vi "continuous-serial-read.vi"() -> ()   [LabVIEW 2021]
uses:
  <vilib>/regexp/Match Regular Expression.xnode
  <vilib>/Instr/_visa.llb/VISA Configure Serial Port (Instr).vi
  SCD41.ctl
  STC31.ctl
panel:
  in  "state":string
  out "CD5":T1 {"CD3: CO2 (ppm)" format="%.2f"}
  out "CD4":T1 {"CD3: CO2 (ppm)" format="%.2f"}
  out "CD3":T1 {"CD3: CO2 (ppm)" format="%.2f"}
  out "CD2":T2 {"Humidity (%)" format="%.2f"; "Temp (degC)" format="%.2f"; "CO2 (ppm)" format="%.2f"}
  out "CD1":T2 {"Humidity (%)" format="%.2f"; "Temp (degC)" format="%.2f"; "CO2 (ppm)" format="%.2f"}
  out "RHT6: Humidity (%)":dbl format="%.2f"
  out "RHT6: Temp (degC)":dbl format="%.2f"
  out "RHT5: Humidity (%)":dbl format="%.2f"
  out "RHT5: Temp (degC)":dbl format="%.2f"
  out "RHT4: Humidity (%)":dbl format="%.2f"
  out "RHT4: Temp (degC)":dbl format="%.2f"
  out "RHT3: Humidity (%)":dbl format="%.2f"
  out "RHT3: Temp (degC)":dbl format="%.2f"
  out "Num Samples":i32
  out "error out":errorcluster
  out "data string array":string[](array[string])
  out "read buffer":string
  out "Bytes Returned":u32
  in  "VISA resource name":refnum<visa-resource-name>="COM22"
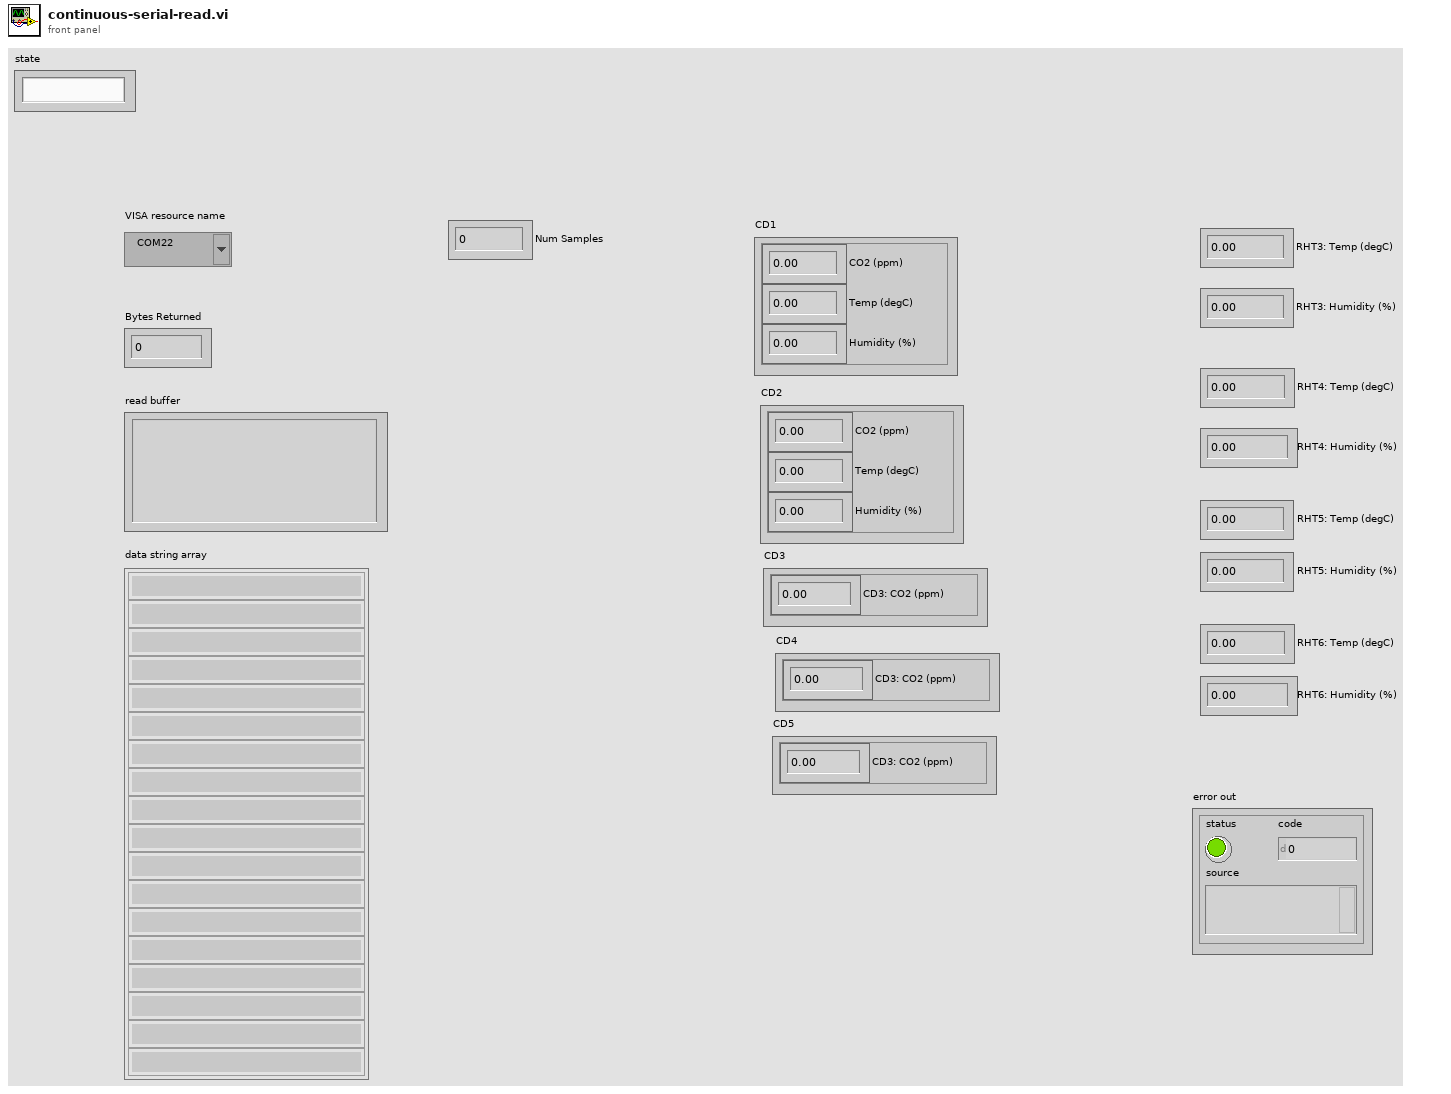
[diagram p1: front panel]
types:
  T1 = typedef "STC31.ctl" = cluster{"CD3: CO2 (ppm)":dbl}
  T2 = typedef "SCD41.ctl" = cluster{"CO2 (ppm)":dbl, "Temp (degC)":dbl, "Humidity (%)":dbl}
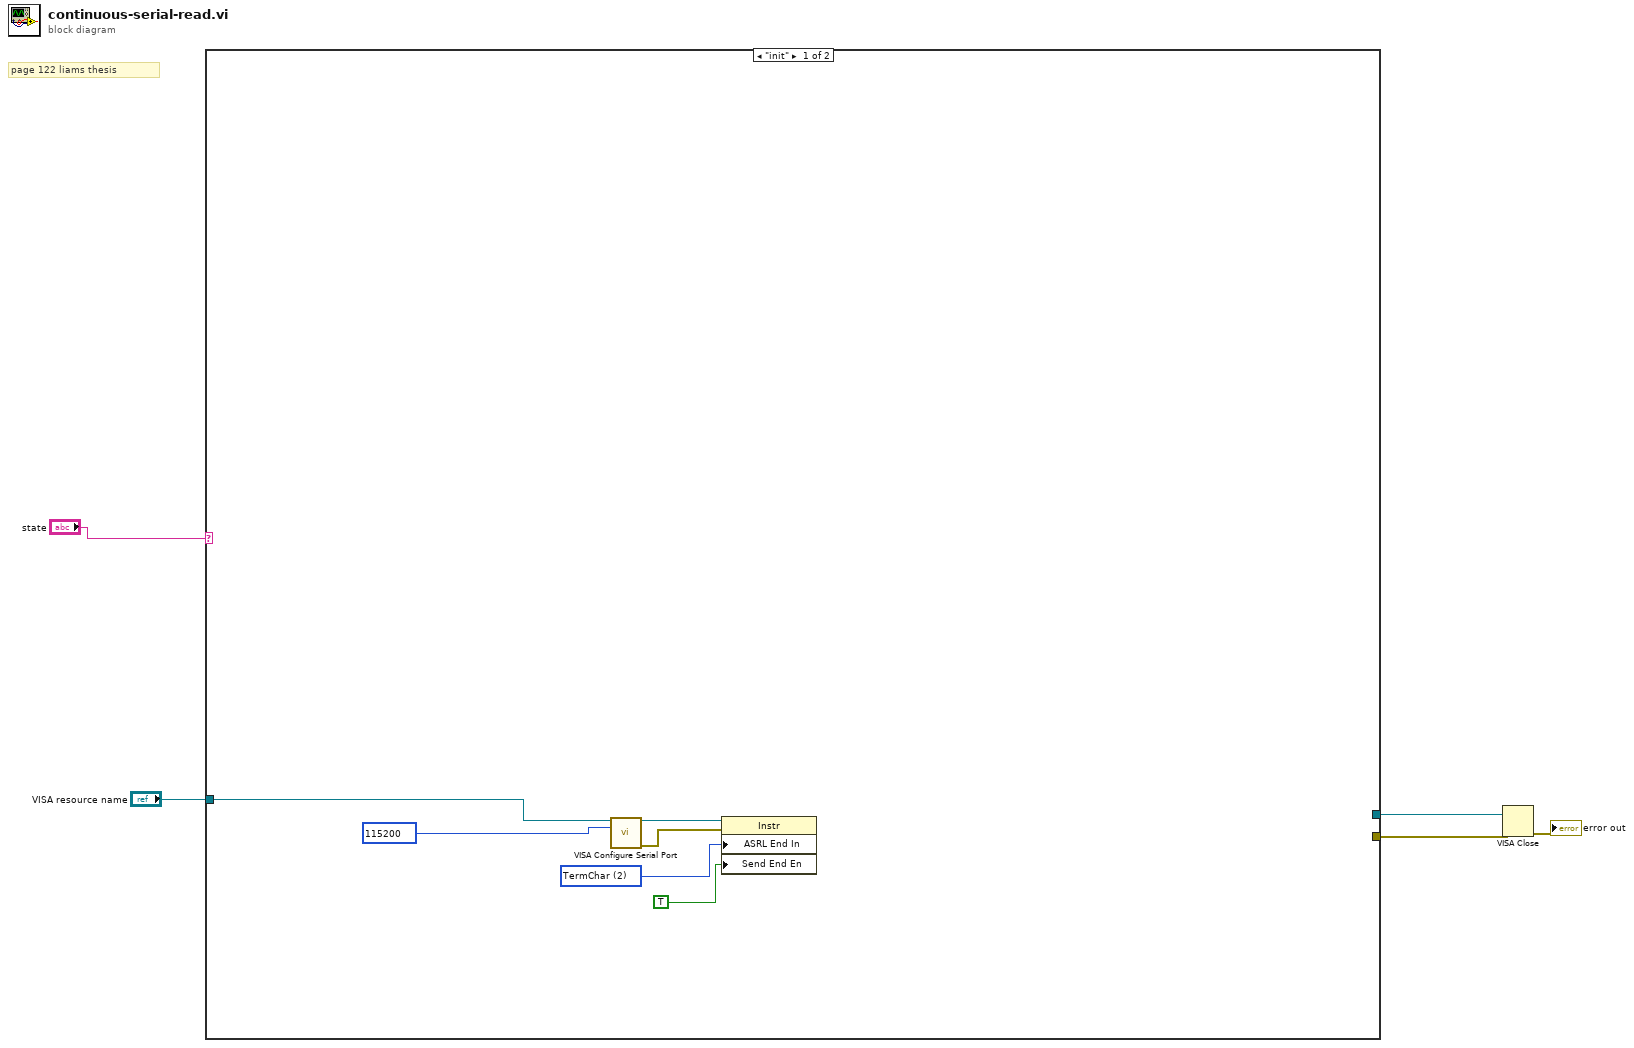
[diagram p0: block diagram]
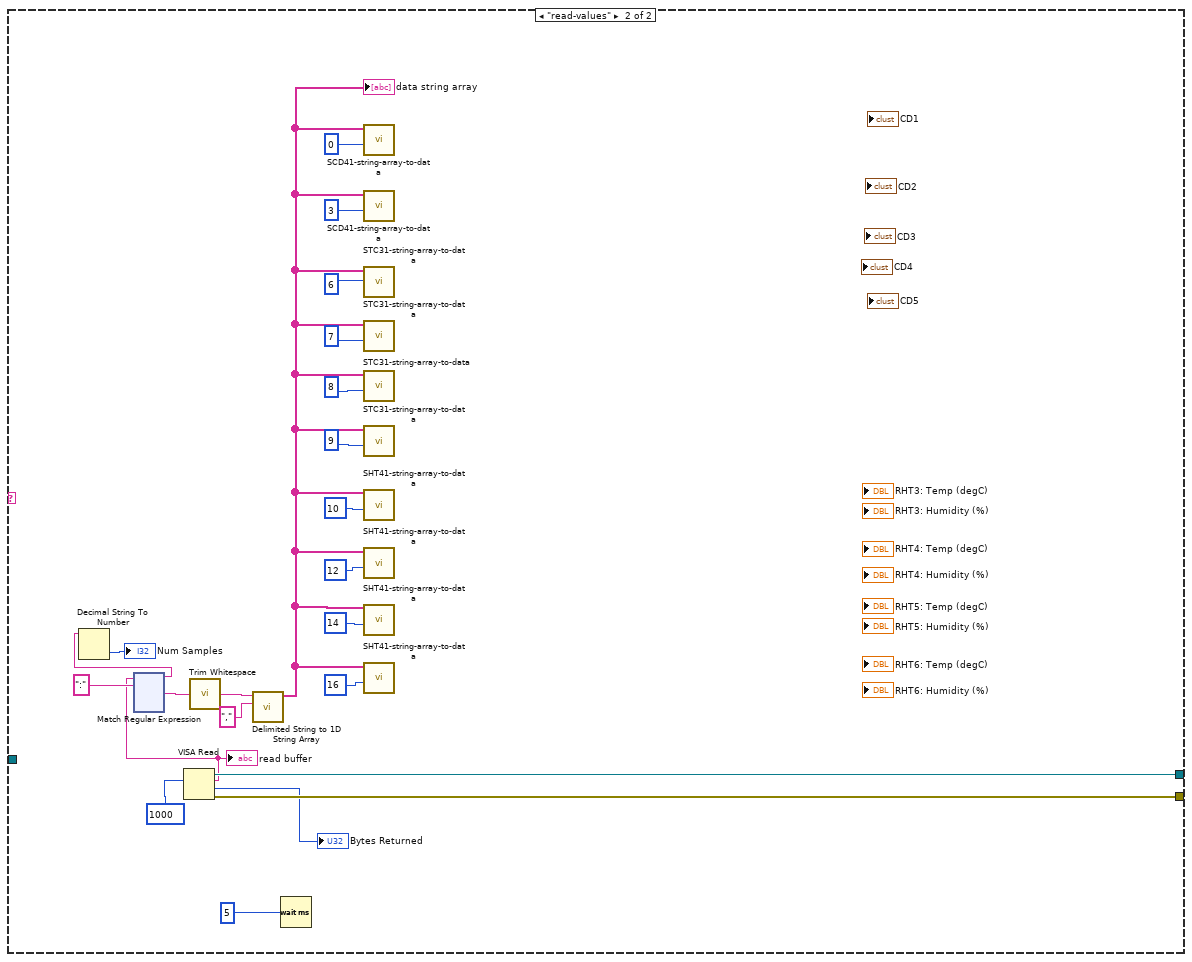
[diagram p2: hidden frame]
diagram:
  # "page 122 liams thesis"
  n1 = case shown="\"init\"" "state" {
    tunnel: [_ w51] -> w5
    tunnel: [_ w50] -> w4
    tunnel: "VISA resource name" -> [w6 _]
    frame "init" {
      w9 = u16 2 items=["None", "Last Bit", "TermChar"] ("Serial Settings:End Mode for Reads")
      n2 = call-poly "VISA Configure Serial Port"("VISA resource name"=w6, "baud rate (9600)"=u32 115200) -> ("VISA resource name out"=w10:refnum<visa-resource-name>, "error out"=w11:errorcluster)  [unwired: 12 in]
      n3 = property class="Instr"(reference=w10, error in=w11, "ASRL End In"=w9, "Send End En"=TRUE ("Message Based Settings:Send End Enable")) -> ()  [unwired: 2 out]
    }
    frame "read-values" {
      n4 = VISA Read(byte count=u32 1000) -> (VISA resource name=w53:refnum<visa-resource-name>, error in (no error)=w52:errorcluster, VISA resource name out=w50:refnum<visa-resource-name>, read buffer=w44:string, return count=→"Bytes Returned":u32, error out=w51:errorcluster)
      "read buffer" <- w44
      n5 = xnode "Match Regular Expression"("input string"=w44, "regular expression"=":" ("delimiter")) -> ("before match"=w43:string, "after match"=w41:string)  [unwired: 4 in, 3 out]
      n6 = Decimal String To Number(string=w43) -> (number=→"Num Samples":i32)  [unwired: 2 in, 1 out]
      n7 = call <vilib>:"Trim Whitespace.vi"("string"=w41) -> ("trimmed string"=w40:string)  [unwired: 1 in]
      n8 = call <vilib>:"Delimited String to 1D String Array.vi"("delimiter"=",", "delimited string"=w40) -> ("string array"=w13:string[])  [unwired: 9 in]
      "data string array" <- w13
      n9 = Wait (ms)(milliseconds to wait=u32 5) -> ()  [unwired: 1 out]
      n10 = call "SCD41-string-array-to-data.vi"("Starting Index"=0, "Data In (string array)"=w13) -> ("SCD41: Humidity (%)"=w26:dbl, "SCD41: Temp (degC)"=w39:dbl)  [unwired: 7 in, 1 out]
      n11 = call "SCD41-string-array-to-data.vi"("Starting Index"=3, "Data In (string array)"=w13) -> ("SCD41: Humidity (%)"=w36:dbl, "SCD41: Temp (degC)"=w12:dbl, "SCD41: CO2 (ppm)"=w37:dbl)  [unwired: 7 in]
      n12 = call "STC31-string-array-to-data.vi"("Starting Index"=6 ("index"), "Data In (string array)"=w13) -> ("STC31: CO2 (ppm)"=w33:dbl)  [unwired: 8 in, 1 out]
      n13 = call "STC31-string-array-to-data.vi"("Starting Index"=7, "Data In (string array)"=w13) -> ("STC31: CO2 (ppm)"=w32:dbl)  [unwired: 8 in, 1 out]
      n14 = call "STC31-string-array-to-data.vi"("Starting Index"=8, "Data In (string array)"=w13) -> ("STC31: CO2 (ppm)"=w31:dbl)  [unwired: 8 in, 1 out]
      n15 = call "STC31-string-array-to-data.vi"("Starting Index"=9, "Data In (string array)"=w13) -> ("STC31: CO2 (ppm)"=w28:dbl)  [unwired: 8 in, 1 out]
      n16 = call "SHT41-string-array-to-data.vi"("Starting Index"=10, "Data In (string array)"=w13) -> ("SHT41: Humidity (%)"=w23:dbl, "SHT41: Temp (degC)"=w24:dbl)  [unwired: 8 in]
      n17 = call "SHT41-string-array-to-data.vi"("Starting Index"=12, "Data In (string array)"=w13) -> ("SHT41: Humidity (%)"=w20:dbl, "SHT41: Temp (degC)"=w21:dbl)  [unwired: 8 in]
      n18 = call "SHT41-string-array-to-data.vi"("Starting Index"=14, "Data In (string array)"=w13) -> ("SHT41: Humidity (%)"=w17:dbl, "SHT41: Temp (degC)"=w18:dbl)  [unwired: 8 in]
      n19 = call "SHT41-string-array-to-data.vi"("Starting Index"=16, "Data In (string array)"=w13) -> ("SHT41: Humidity (%)"=w14:dbl, "SHT41: Temp (degC)"=w15:dbl)  [unwired: 8 in]
    }
  }
  n20 = VISA Close(VISA resource name=w4, error in (no error)=w5) -> (error out=→"error out":errorcluster)
